vi "溶解氧电极校准.vi"() -> ()   [LabVIEW 2016, in "斯坦道多参数.lvlib"]
uses:
  <vilib>/Utility/miscctls.llb/LVPointTypeDef.ctl
  <vilib>/Analysis/NI_AALBase.lvlib
panel:
  out "滤波设定":dbl
  out "标液2":string="饱和标准液"
  out "标液1":string="零点标准液"
  in  "刷新按钮":bool
  out "第二点信号值":dbl
  out "第一点信号值":dbl
  out "通讯状态":string
  out "第二点校准值":dbl
  out "第一点校准值":dbl
  out "最小值":sgl format="%#.2f"
  out "最大值":sgl format="%#.2f"
  in  "校准模式":u16(ring)=1 items=["两点校准", "单点校准"]
  in  "校准停止":bool
  in  "校准启动":bool
  out "波形图表":sgl(graph) caption="历史曲线"
  out "变异系数":dbl format="%#.6f"
  out "standard deviation":dbl caption="标准差" format="%#.2f"
  out "mean":dbl caption="均值" format="%#.2f"
  out "测量读值":dbl caption="测量值" format="%#.2f"
  out "偏移值补偿":dbl caption="溶解氧偏移修正值" format="%#.2f"
  out "饱和度值":dbl format="%#.2f"
  out "提示":string
  out "气压补偿值":dbl format="%#.2f"
  out "盐度补偿值":dbl format="%#.2f"
  out "电极斜率":dbl format="%#.6f"
  out "电极零点":dbl format="%#.6f"
  # "溶解氧电极设定"
  # "%"
  # "%"
  # "ppt"
  # "hPa"
  # "请选择校准模式:"
  # "mg/L"
  # "%"
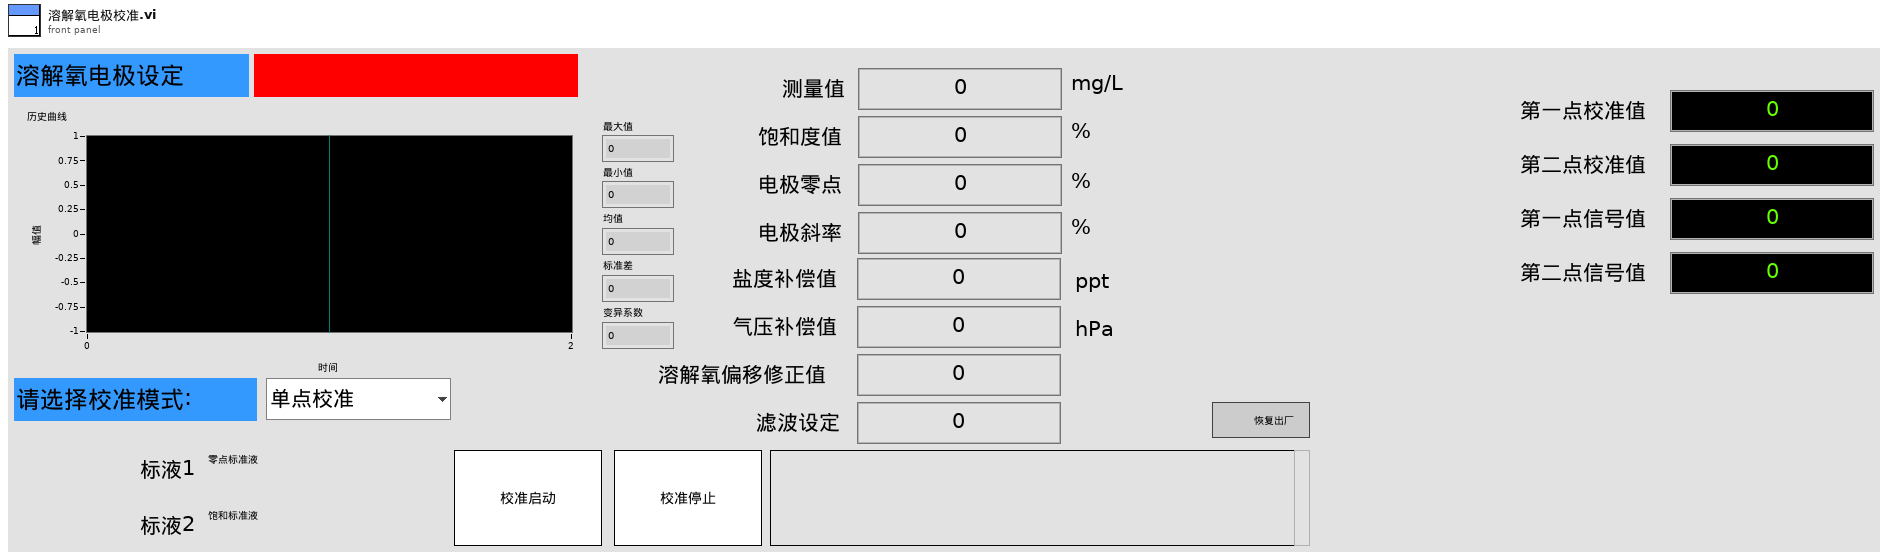
[diagram p1: front panel]
types:
  T1 = typedef "LVPointTypeDef.ctl" = cluster{"Horizontal":i16, "Vertical":i16}
  T2 = cluster{"电极状态标志":u16, "电极型号标志":u16, "溶解氧测量值":sgl, "温度测量值":sgl, "溶解氧饱和度值":sgl, "盐度补偿值":sgl, "大气压补偿值":sgl, "溶解氧偏移修正值":sgl, "温度偏移修正值":sgl, "手动温度补偿值":sgl, "溶解氧电极零点":sgl, "溶解氧电极斜率":sgl, "第1点标准值记录":sgl, "第1点信号值记录":sgl, "第1点温度值记录":sgl, "第2点标准值记录":sgl, "第2点信号值记录":sgl, "第2点温度值记录":sgl, "命令滤波设定":u16, "温度模式":enum16{"ATC", "MTC"}, "生产批次":u16, "电极序号":u16, "串口地址":u16, "串口波特率":enum16{"9600", "19200", "115200"}, "串口校验位":enum16{"NONE", "ODD", "EVEN"}, "串口停止位":enum16{"1bit", "2bit"}, "第一点标准值":sgl, "第二点标准值":sgl}
  T3 = enum8{"Enabled", "Disabled", "Disabled and Grayed Out"}
  T4 = cluster{"测量量程":dbl, "测量精度":dbl, "测量间隔":dbl, "消解温度":dbl, "消解时长":dbl, "空白校准时间":timestamp, "曲线截距":dbl, "曲线斜率":dbl, "测量检出限":dbl, "测量信号值":dbl, "线性相关系数":dbl, "二次多项式系数":dbl, "标样校准时间":timestamp, "单位":enum16{"ug/L", "mg/L"}}
  T5 = cluster{"ph":bool, "DO":bool, "Cond":bool, "Turb":bool, "叶绿素a":bool, "藻密度":bool, "ORP":bool}
  T6 = cluster{"温度测量值":sgl, "测量值":sgl, "温度偏移修正值":sgl, "信号值":sgl}
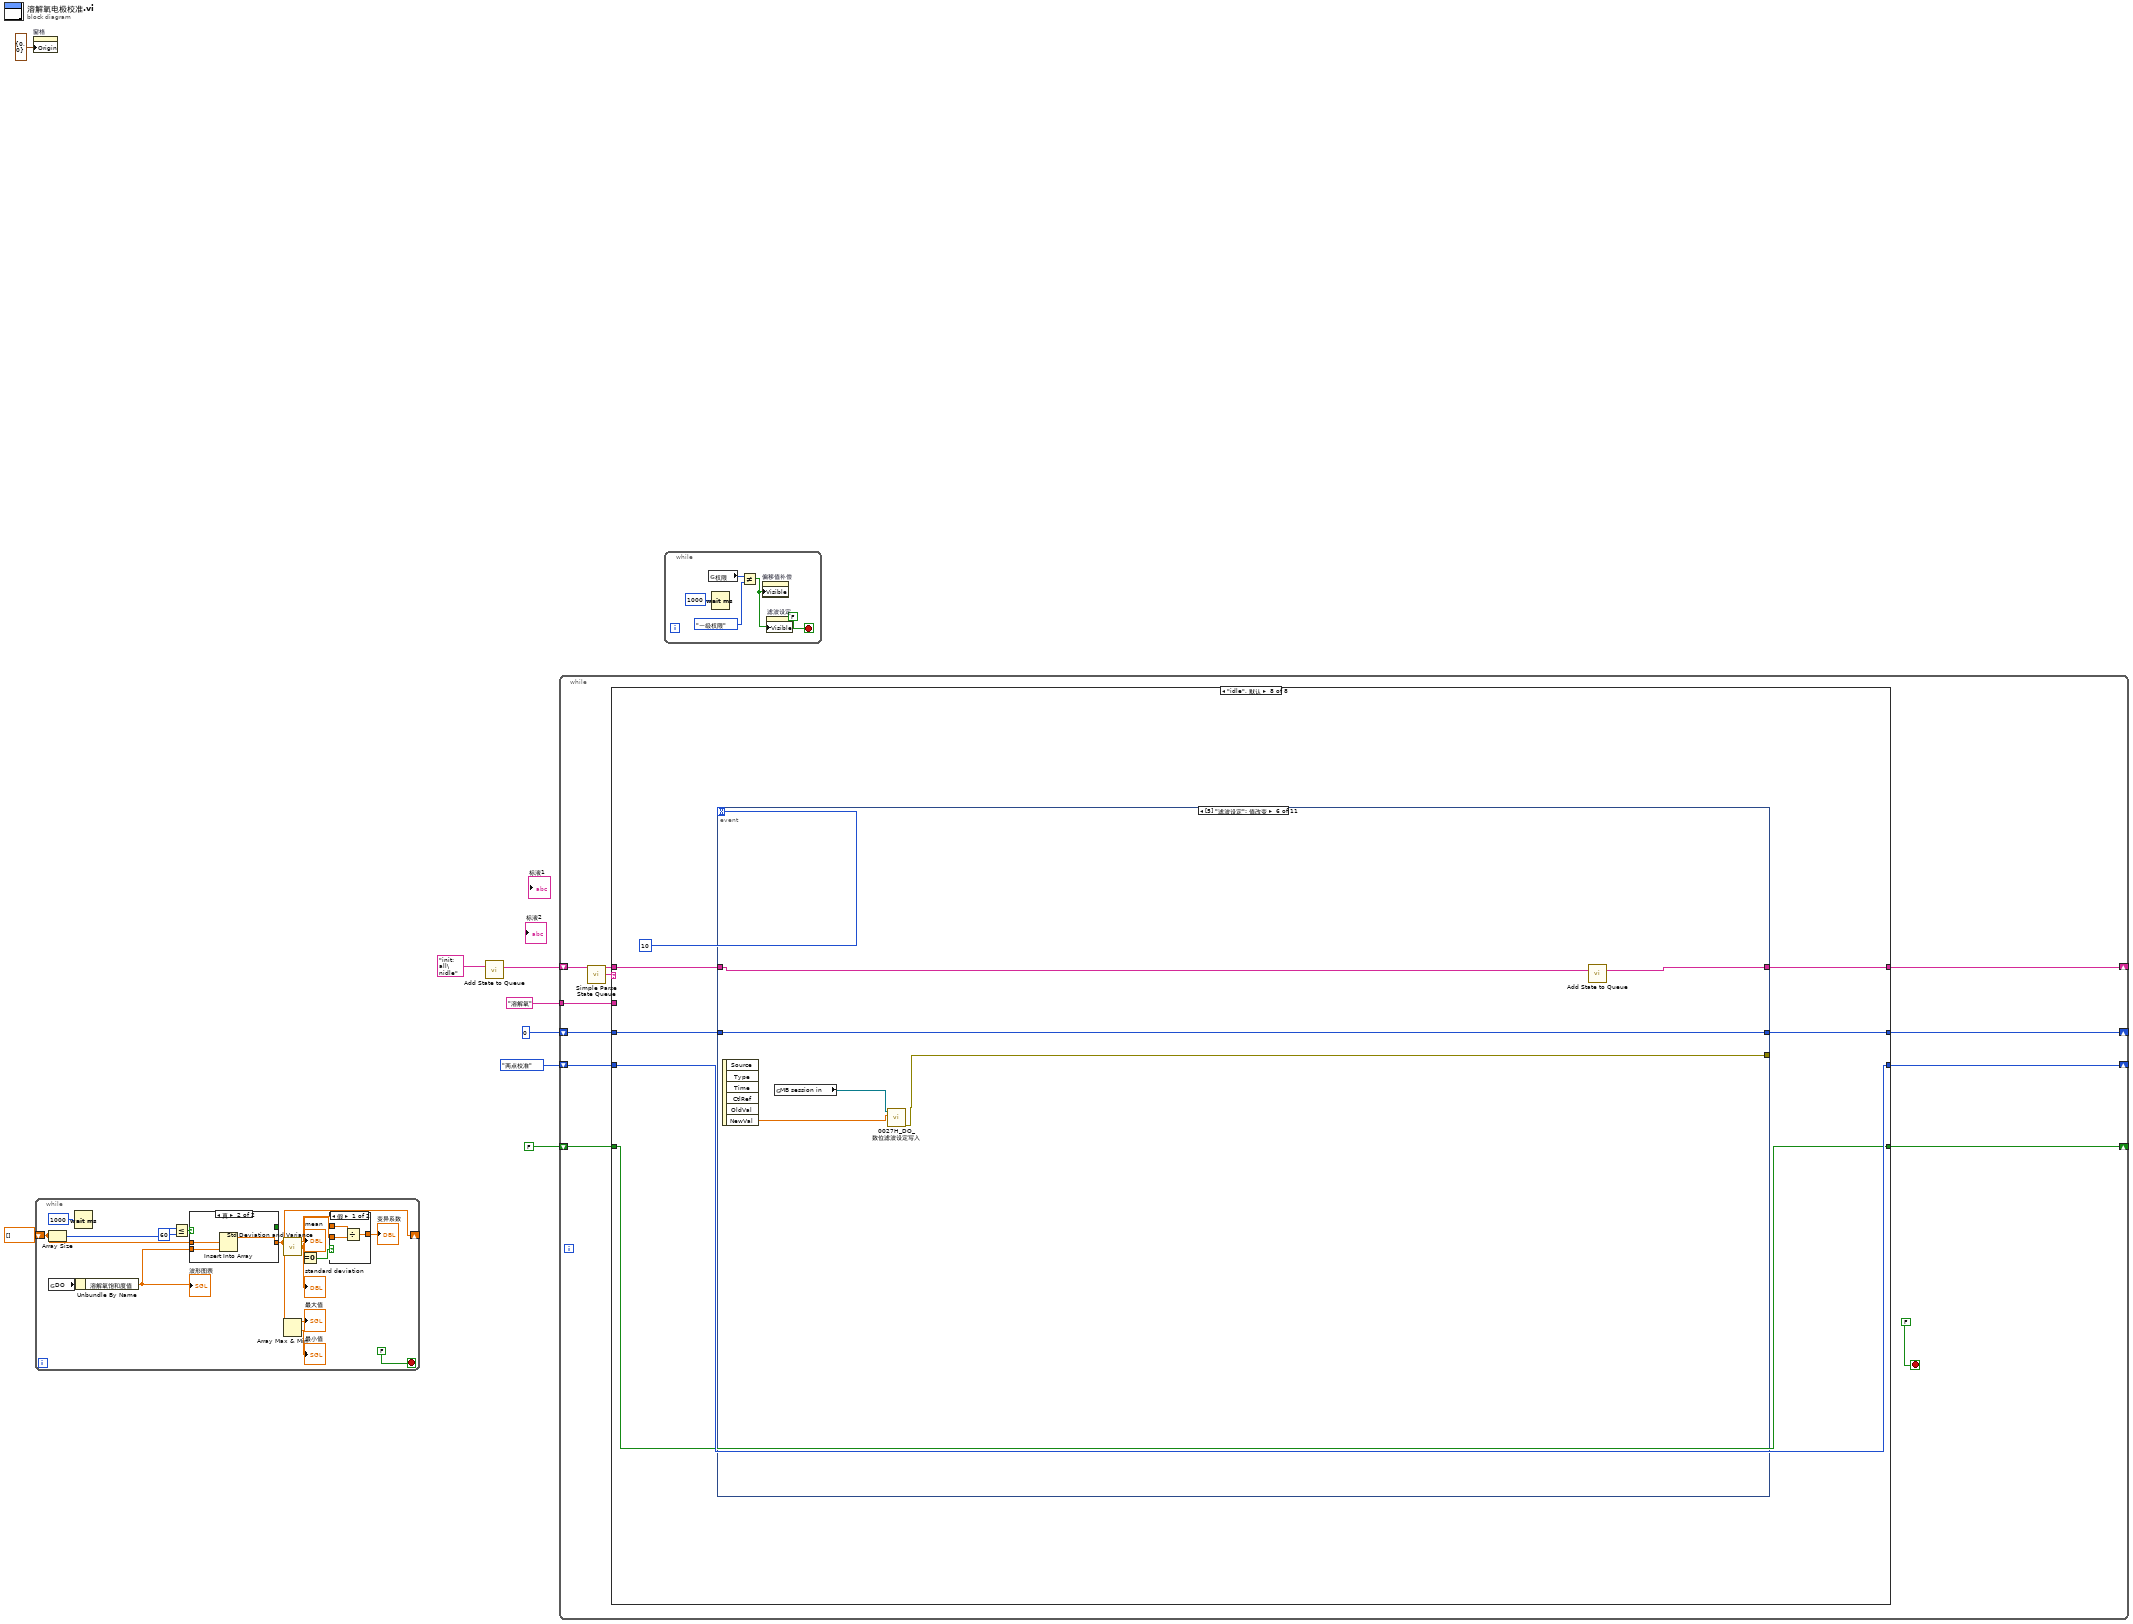
[diagram p0: block diagram]
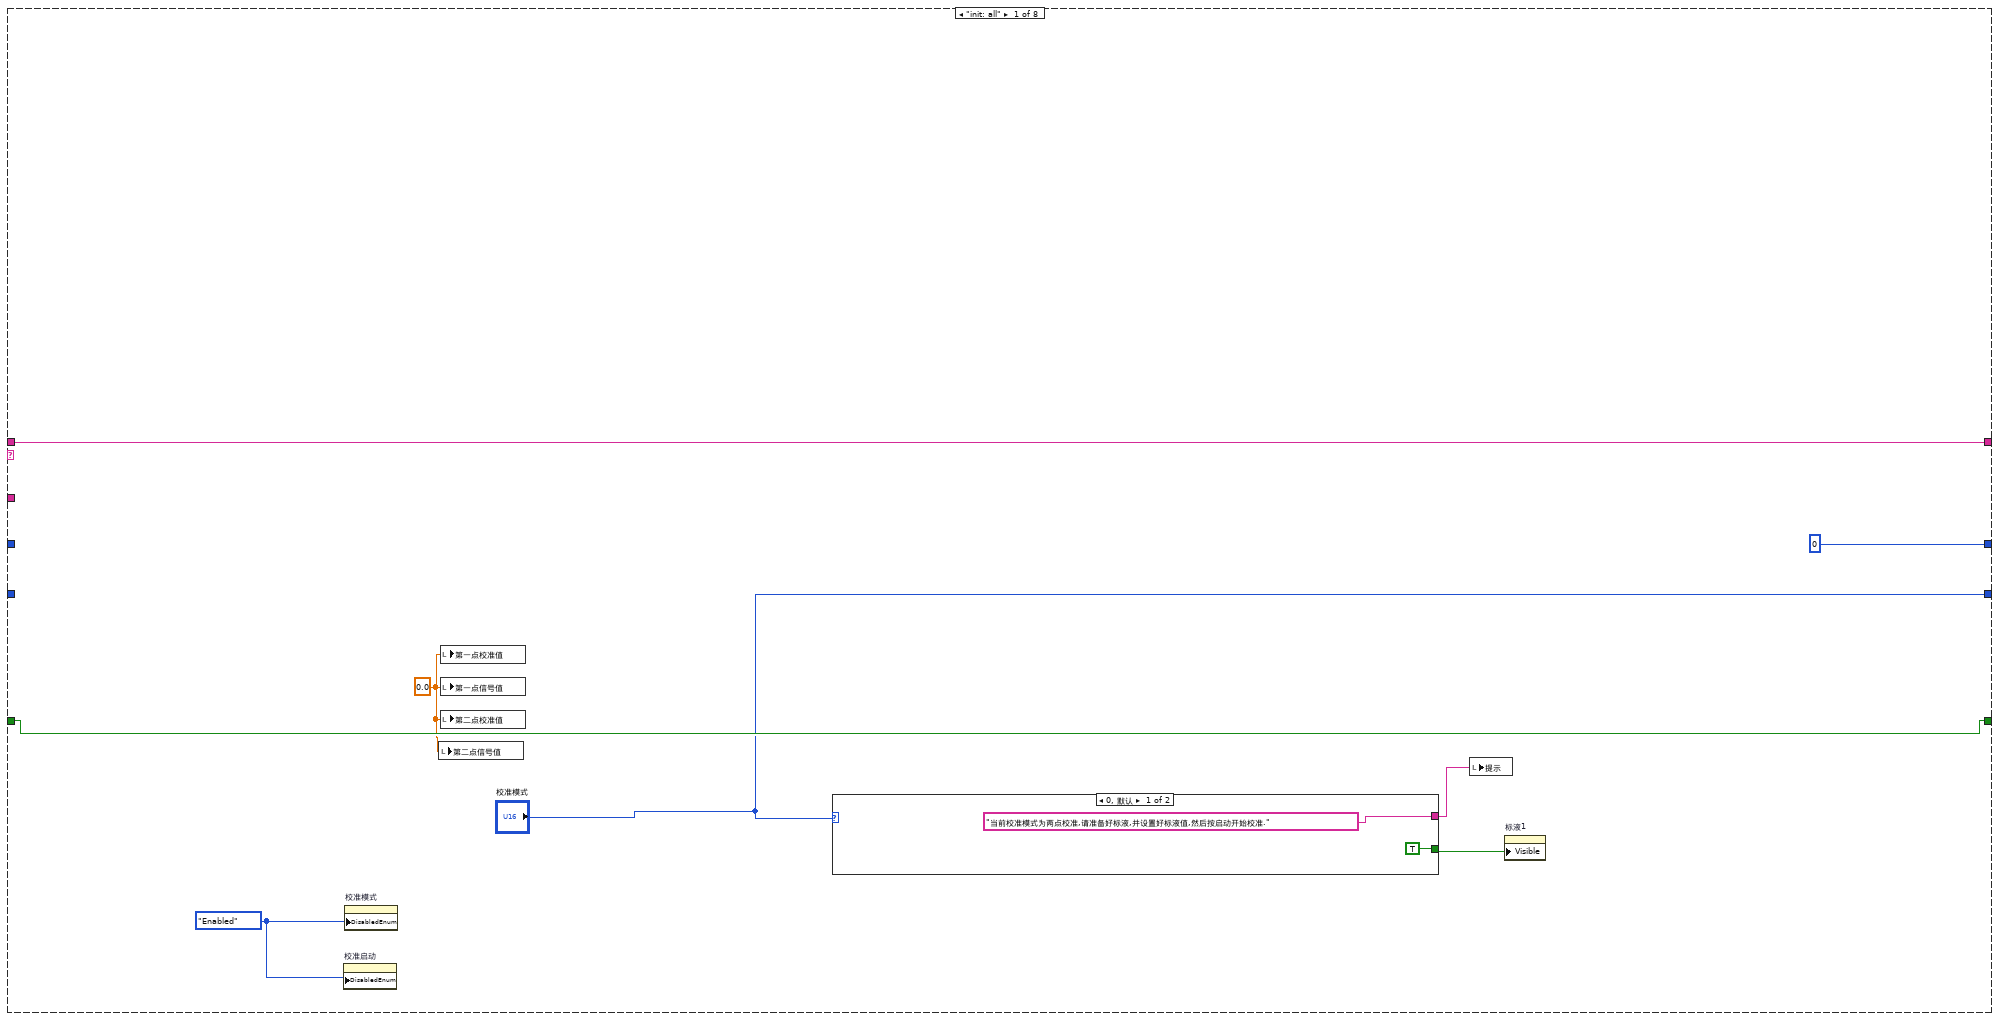
[diagram p2: hidden frame]
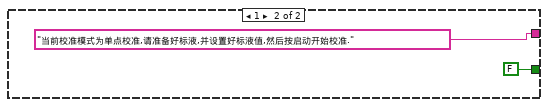
[diagram p3: hidden frame]
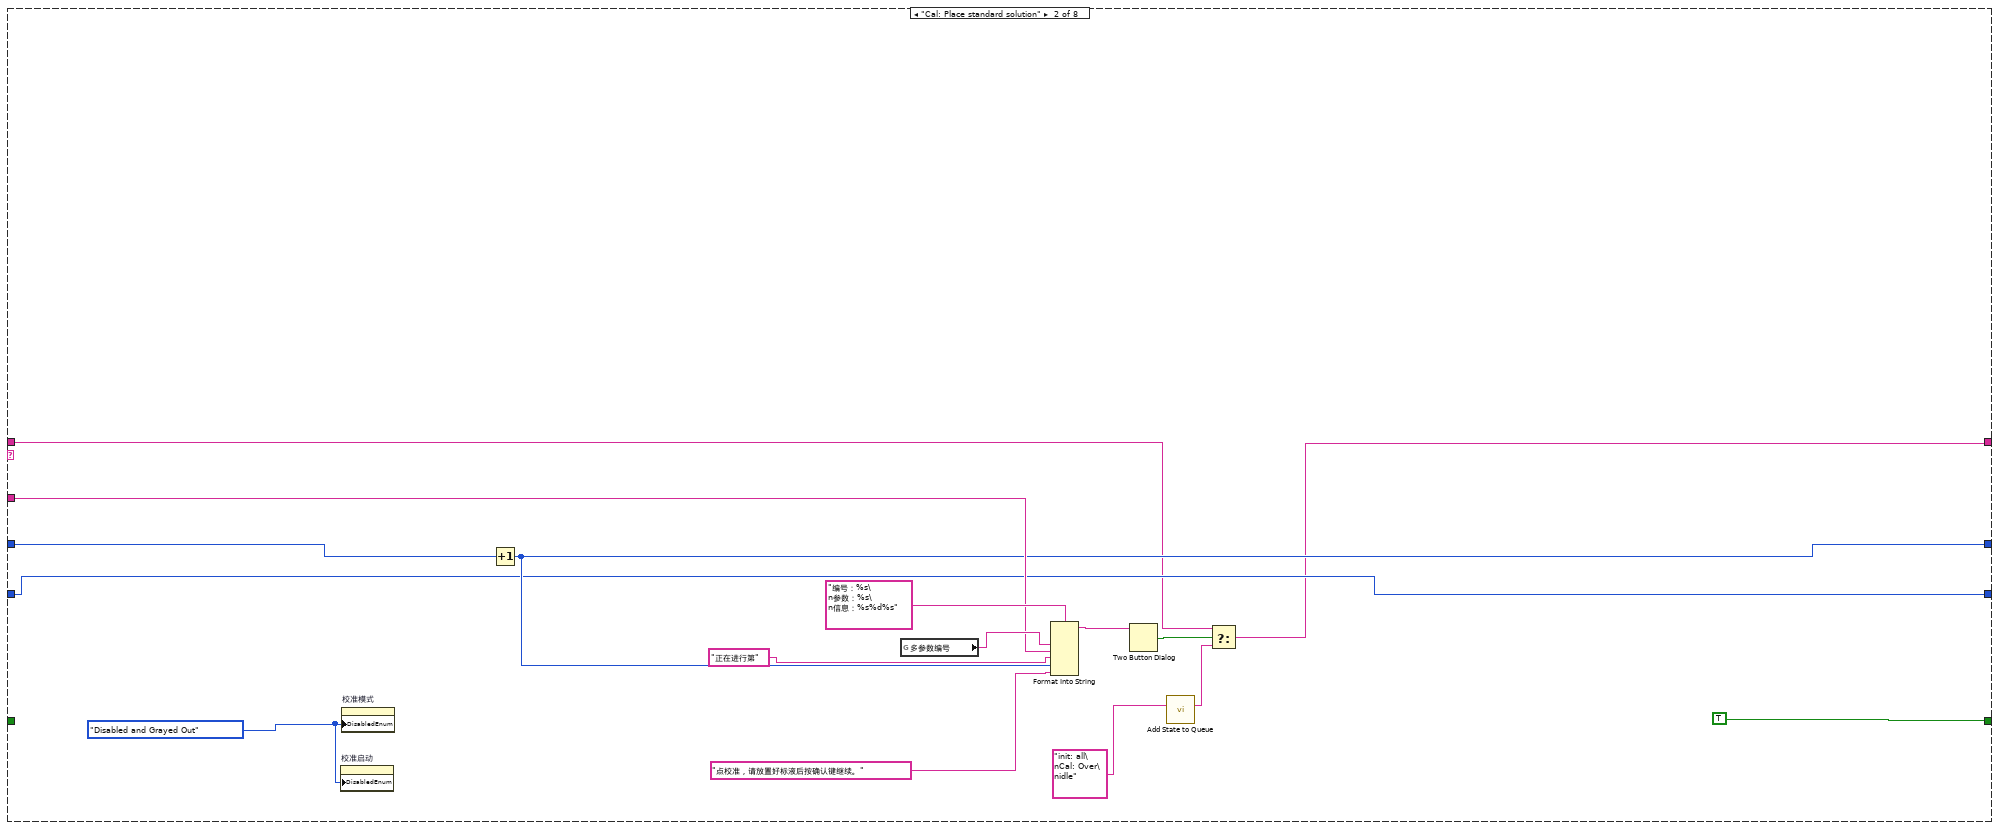
[diagram p4: hidden frame]
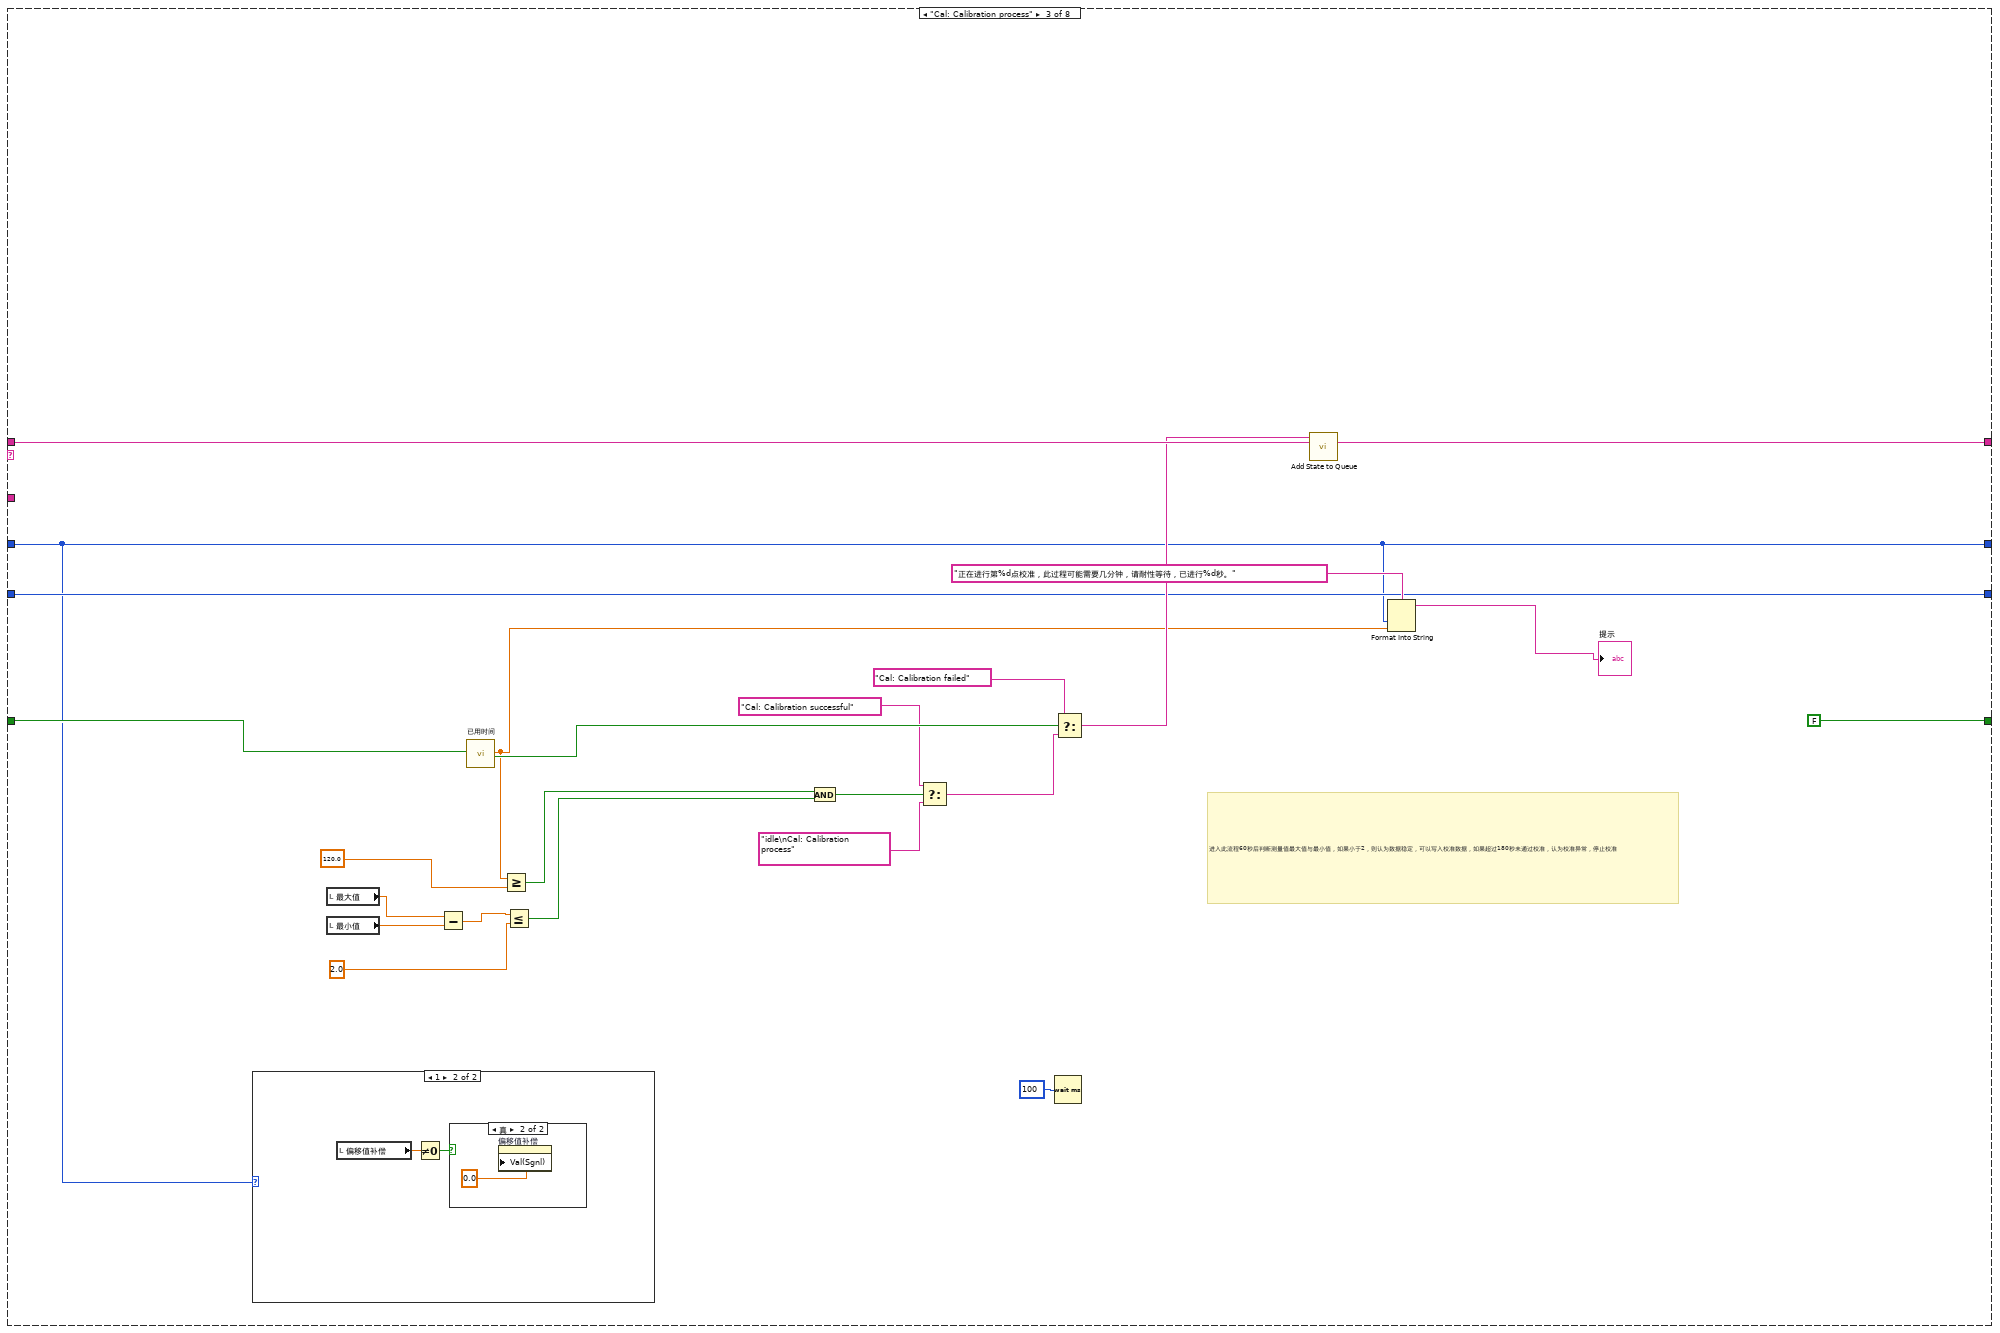
[diagram p5: hidden frame]
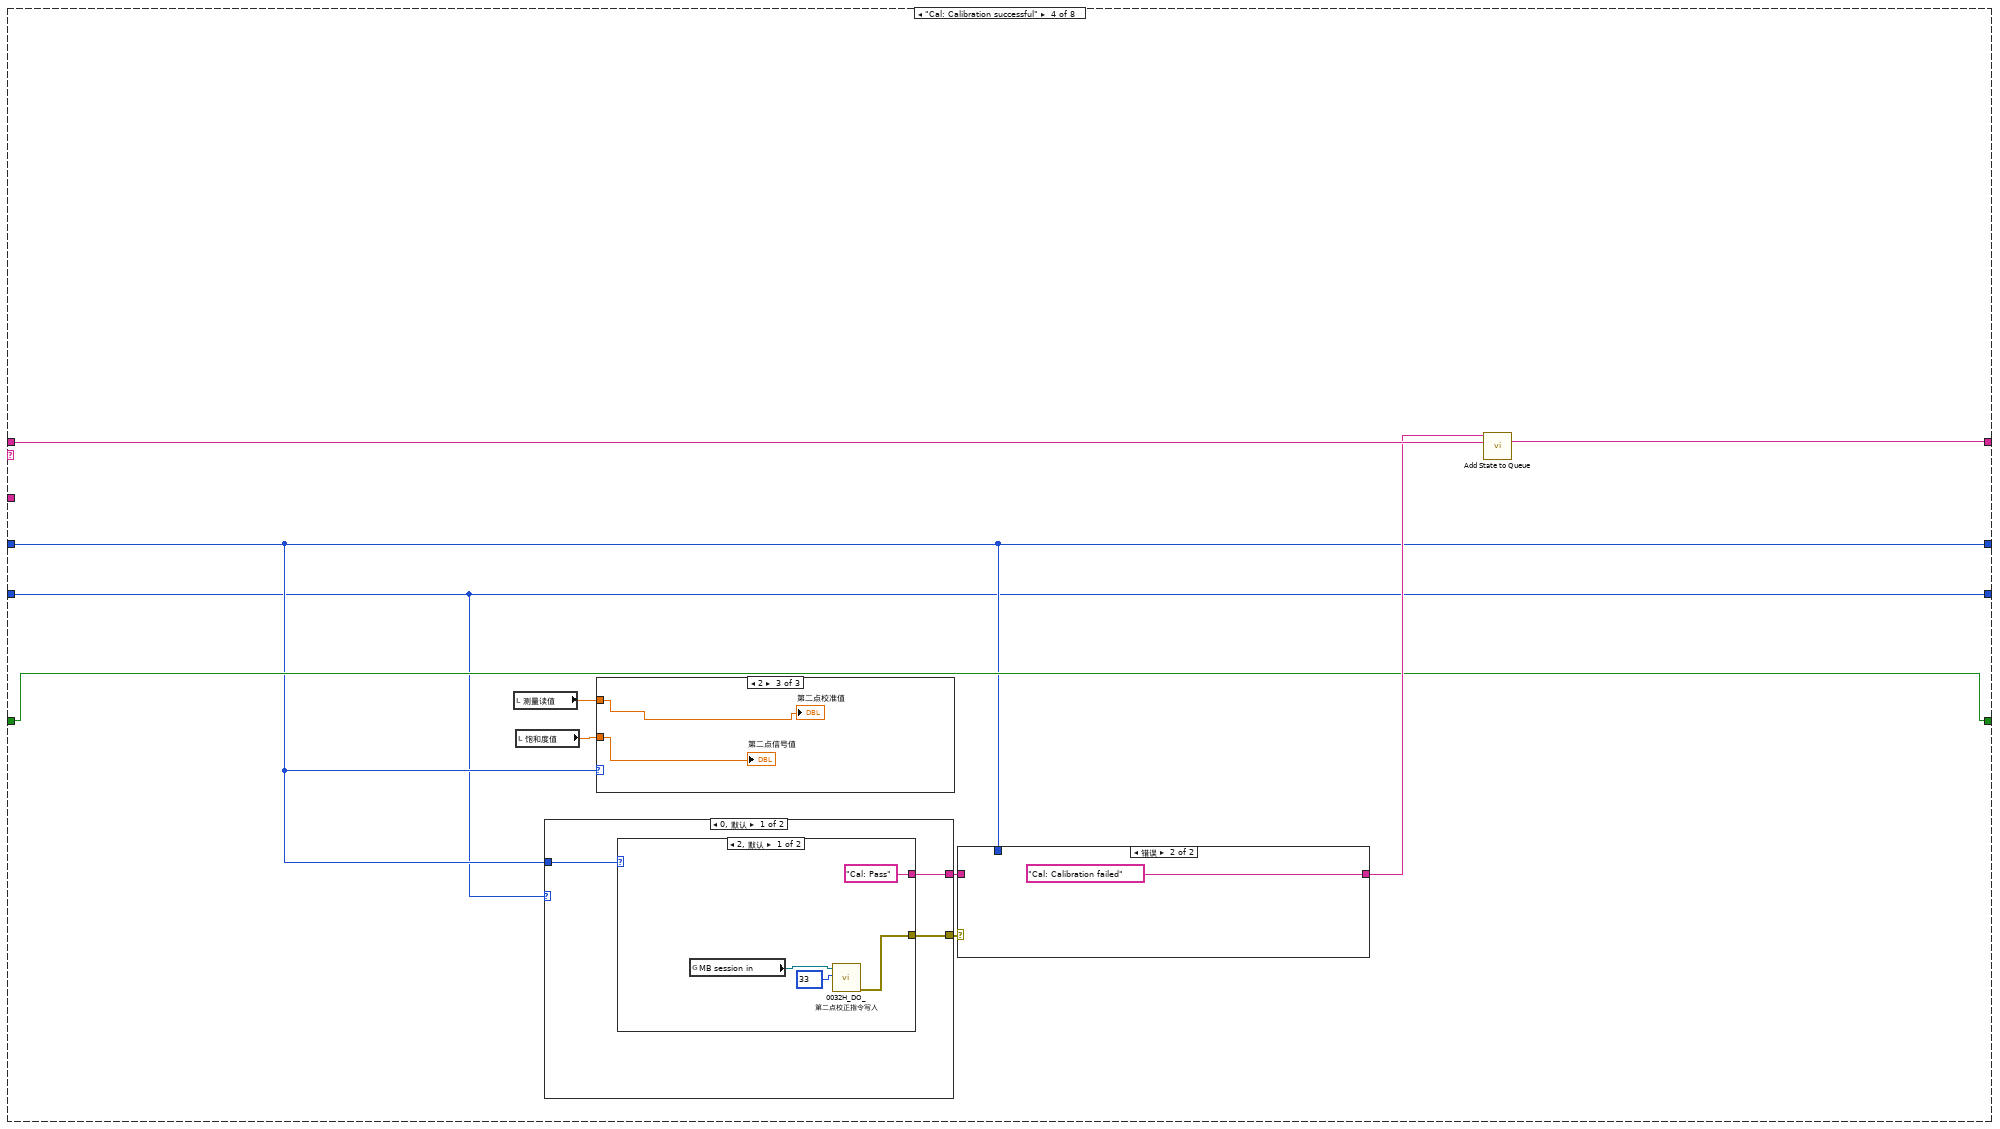
[diagram p8: hidden frame]
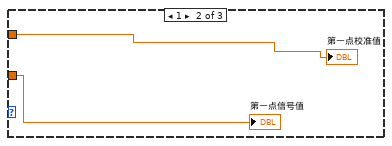
[diagram p10: hidden frame]
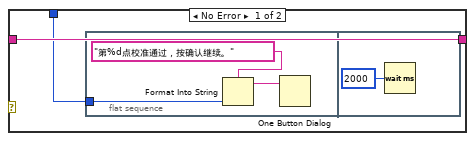
[diagram p11: hidden frame]
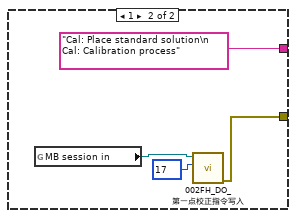
[diagram p12: hidden frame]
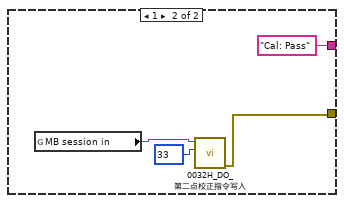
[diagram p13: hidden frame]
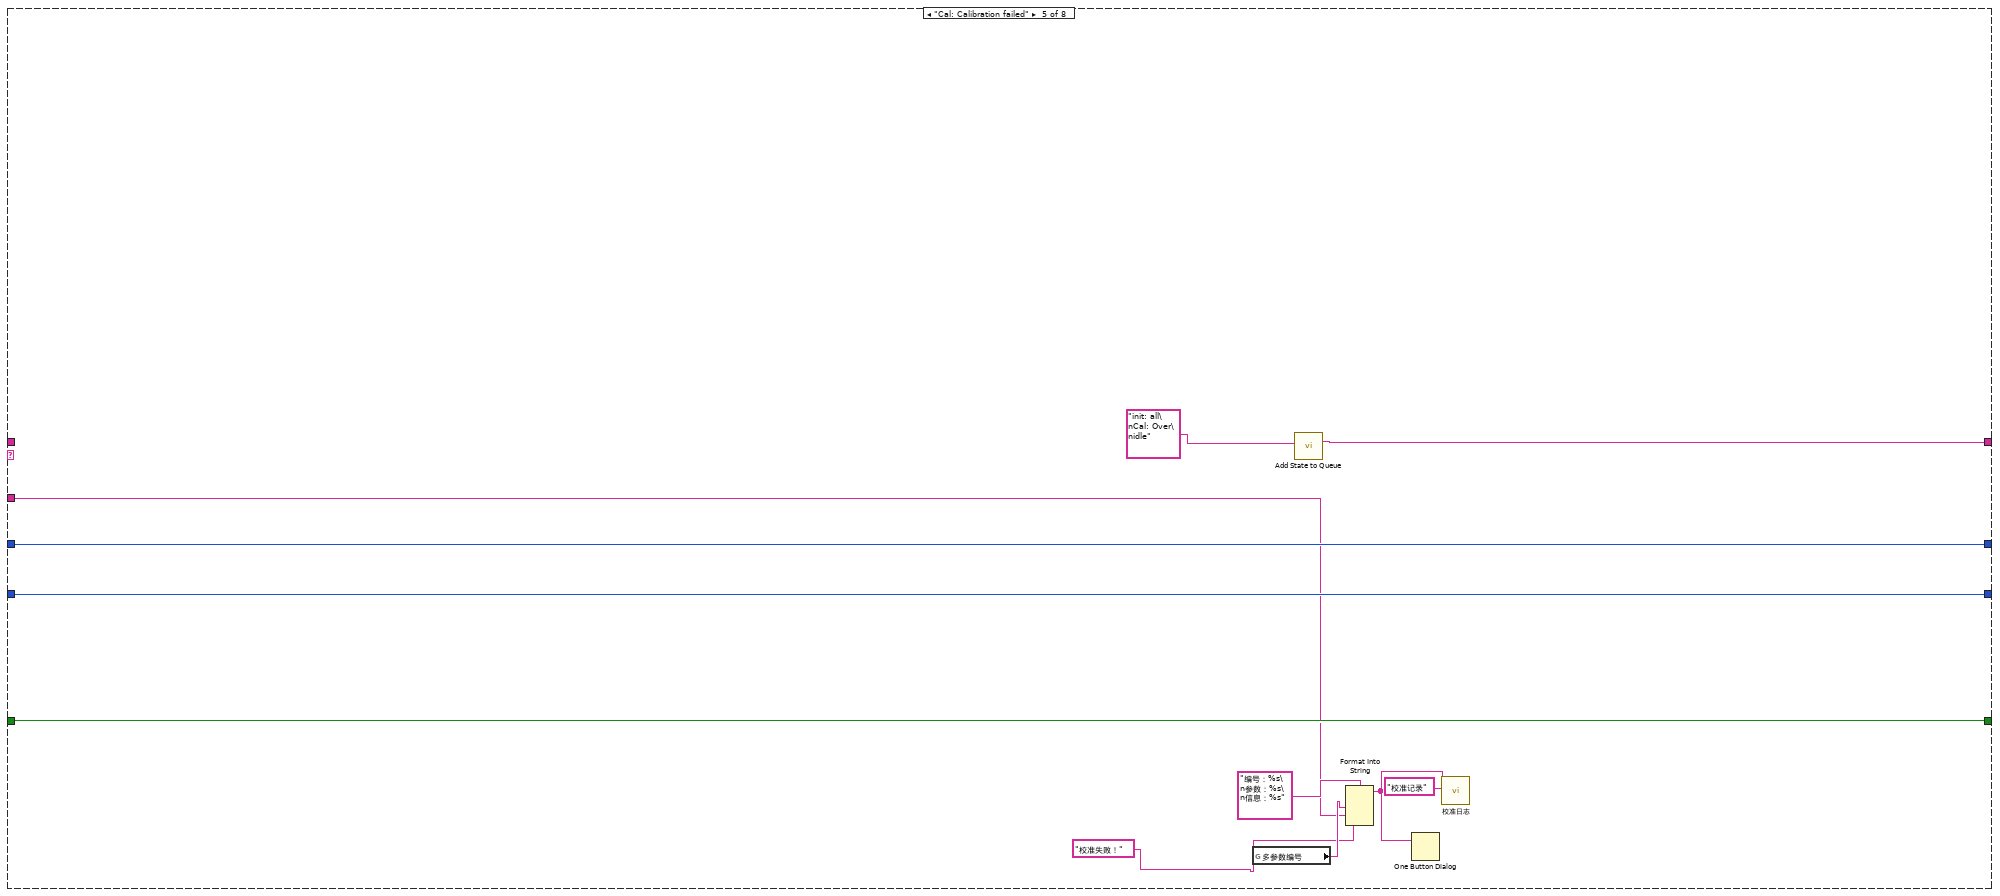
[diagram p14: hidden frame]
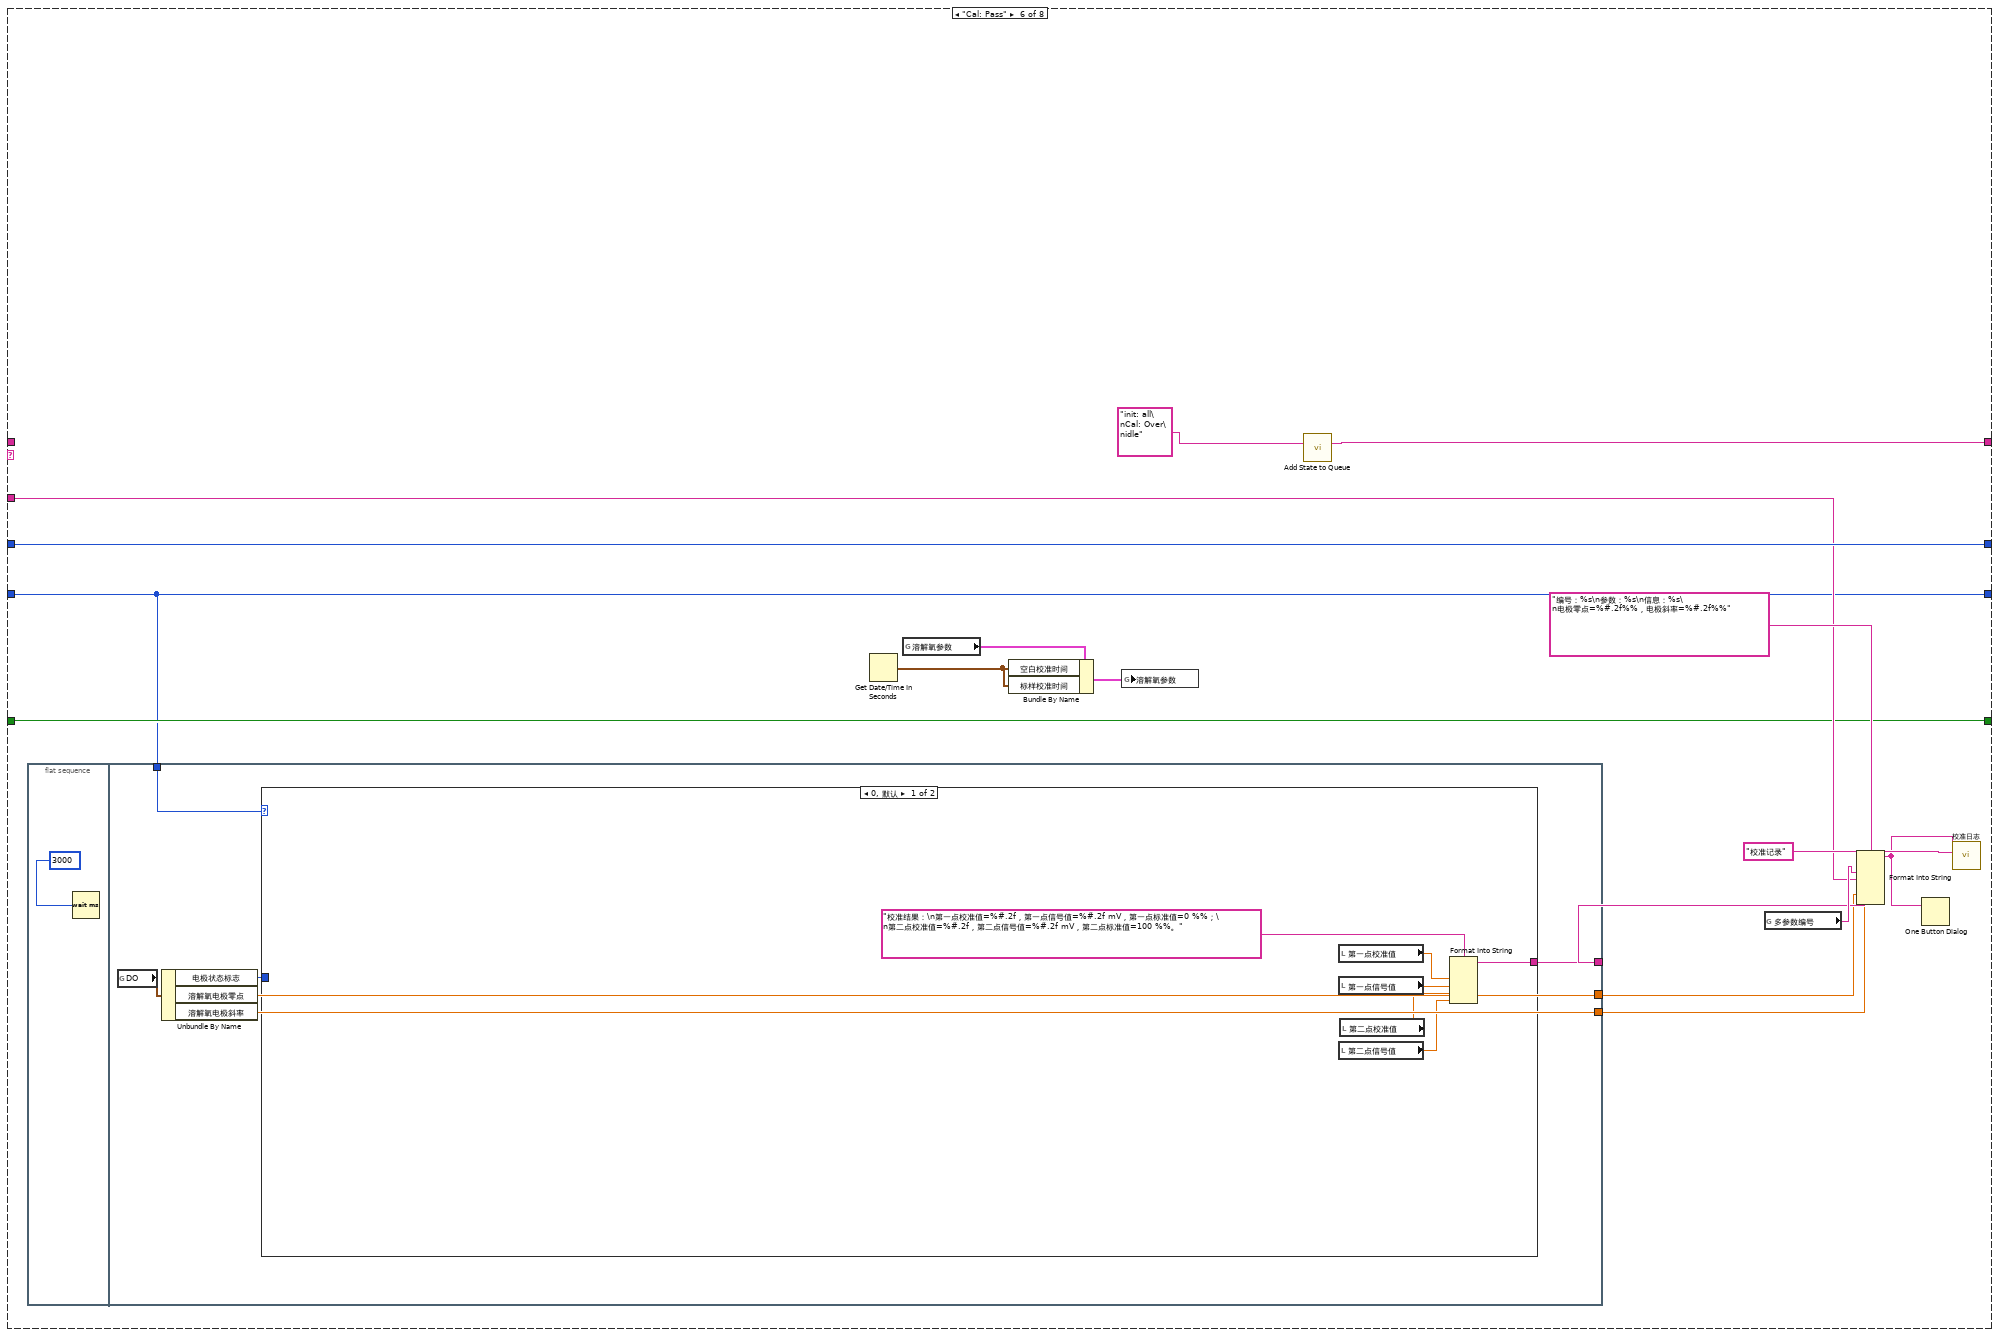
[diagram p15: hidden frame]
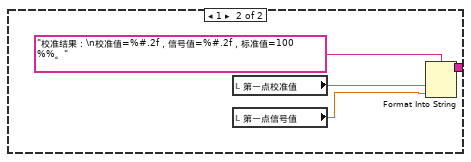
[diagram p16: hidden frame]
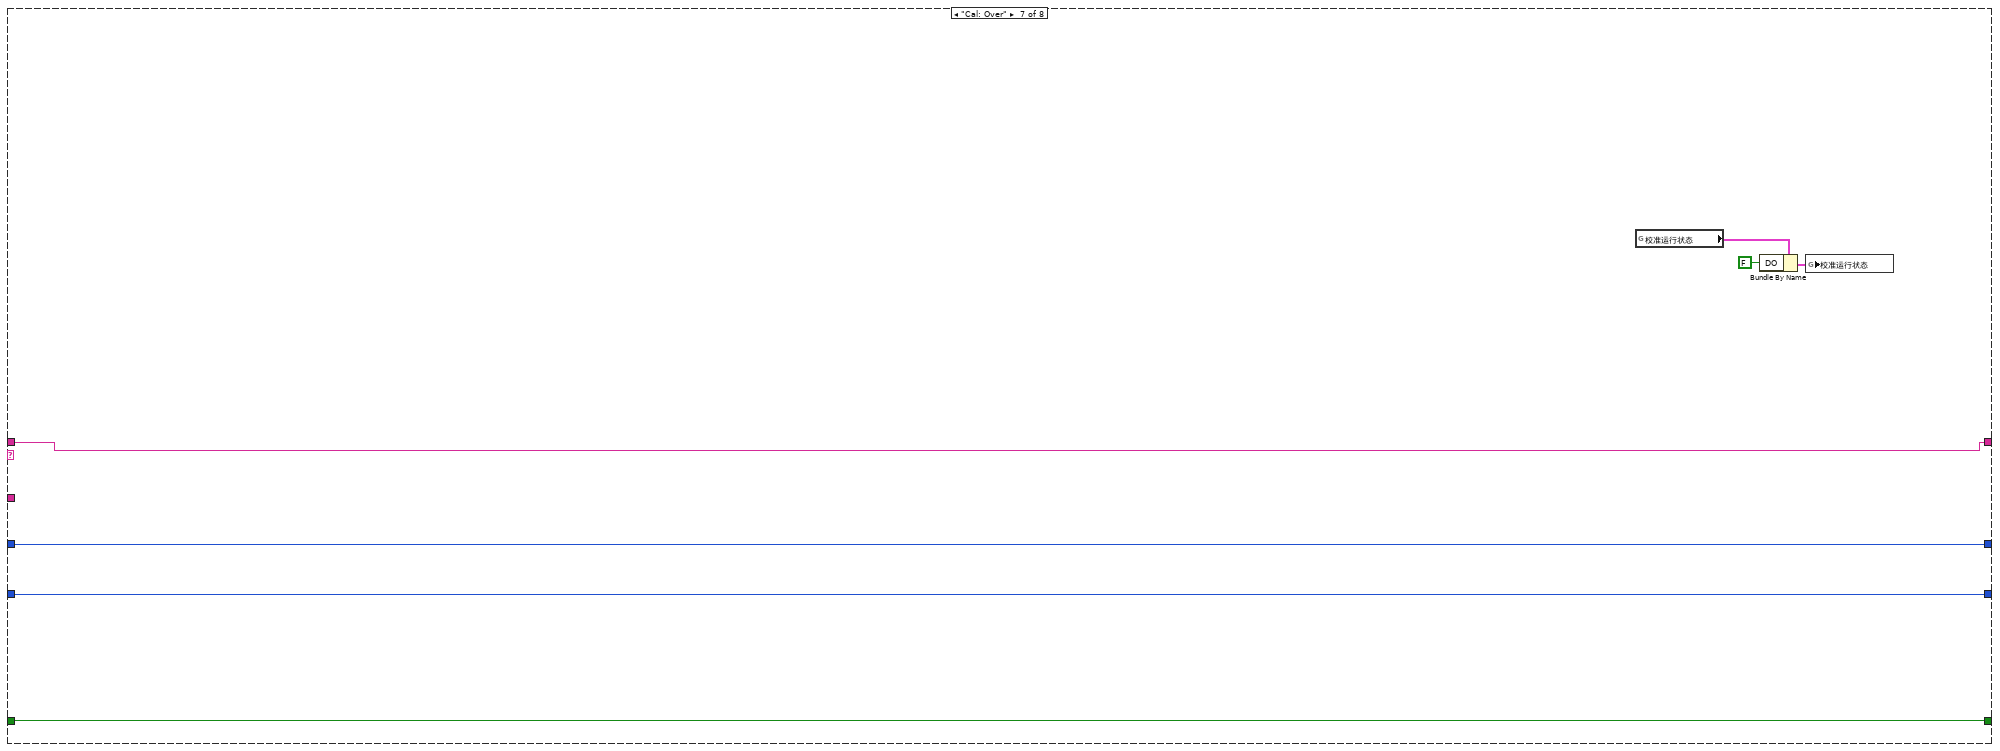
[diagram p17: hidden frame]
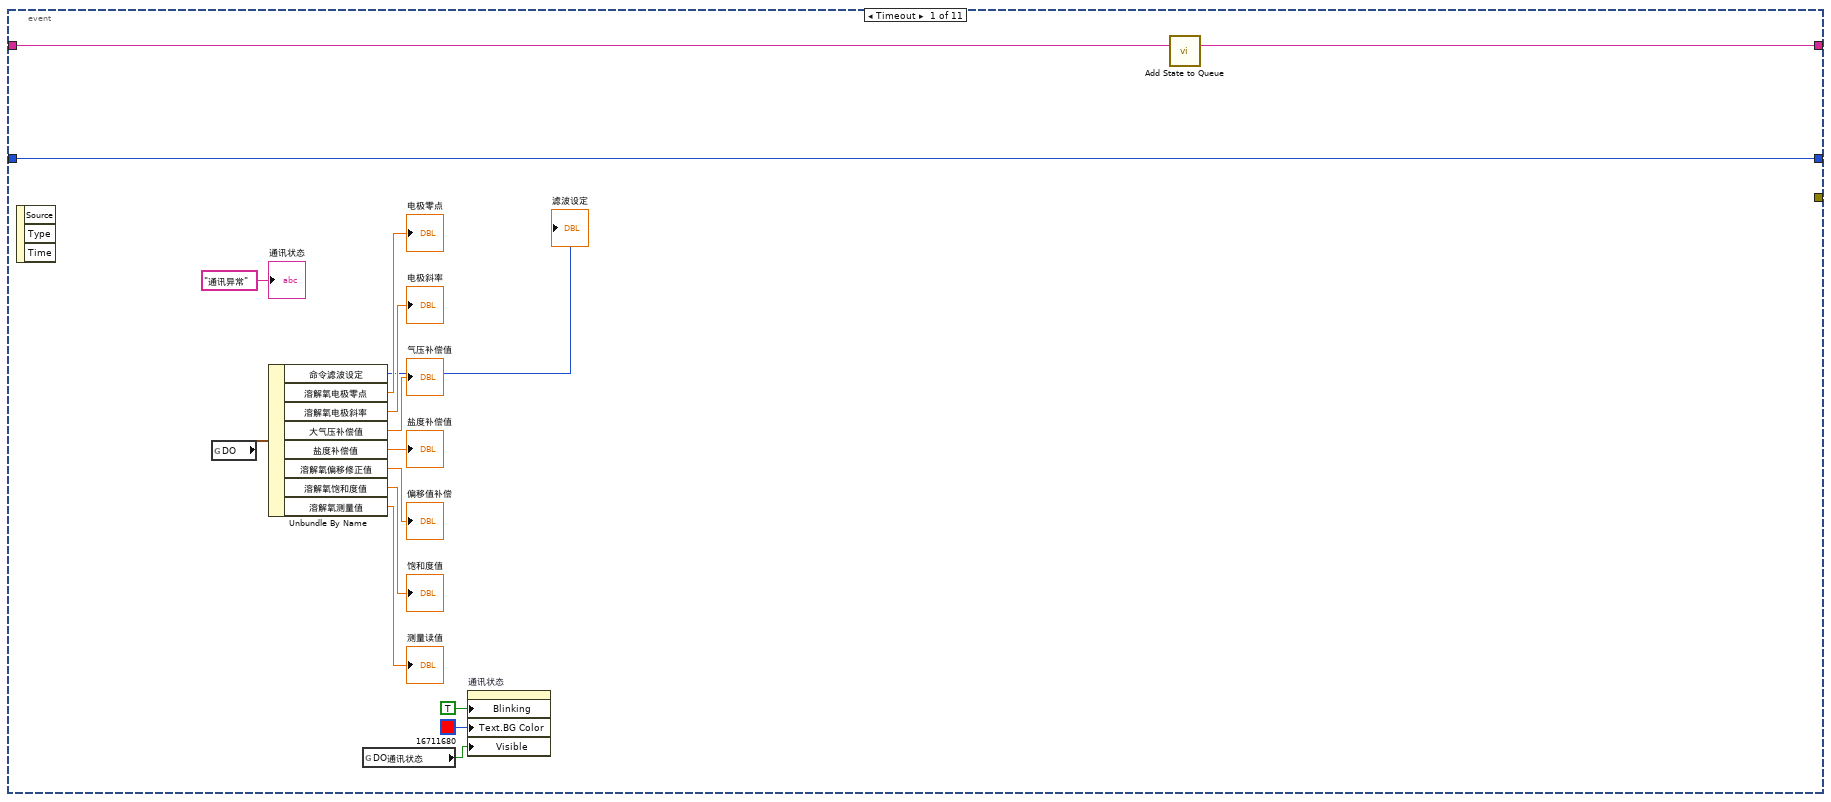
[diagram p18: hidden frame]
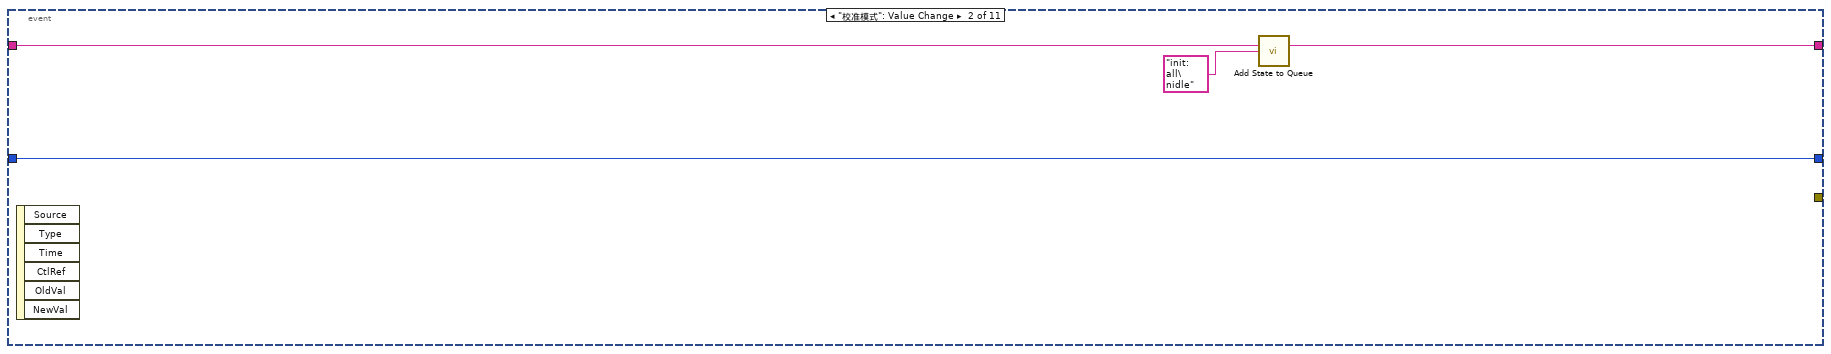
[diagram p19: hidden frame]
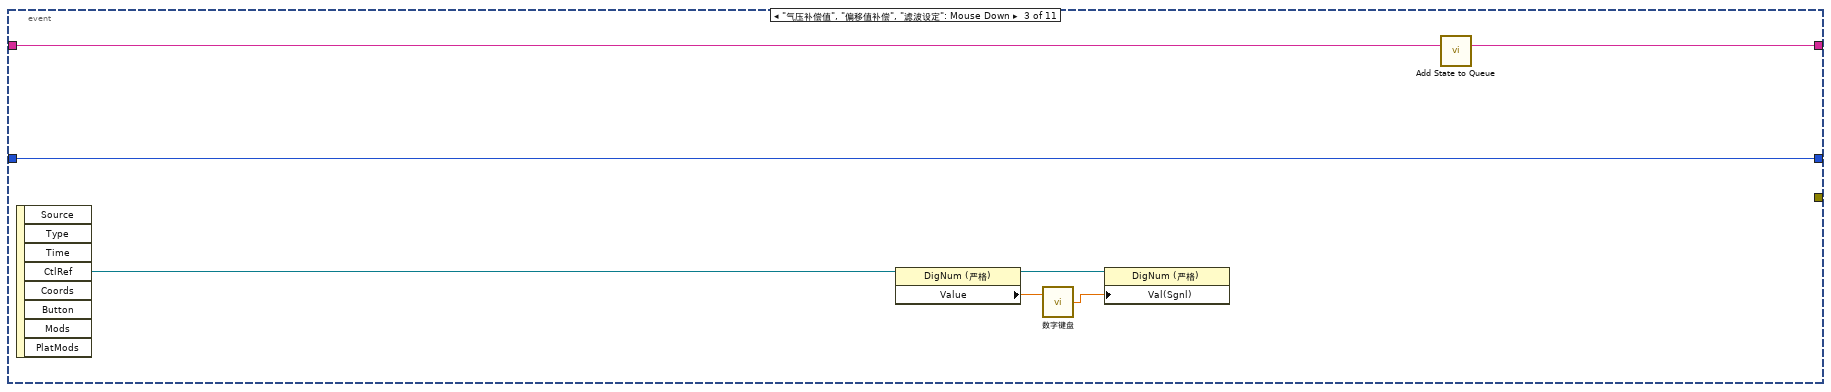
[diagram p20: hidden frame]
diagram:
  n1 = property on="窗格" class="Pane"("Origin"=T1 {"Horizontal"=0, "Vertical"=0} ("原点")) -> ()  [unwired: 2 in, 2 out]
  n2 = while {
    shift-right: [w12] -> _
    shift-left: sgl[] [] -> [w19]
    stop <- FALSE stop-if-true
    n3 = Array Size(array=w19) -> (size(s)=w21:i32)
    n4 = global read "国弘过程全局变量.vi" "DO"() -> (w15:T2)
    n5 = Wait (ms)(milliseconds to wait=u32 1000 ("等待时间（毫秒）")) -> ()  [unwired: 1 out]
    n6 = Unbundle By Name(w15) -> ("溶解氧饱和度值"=w9:sgl)
    "波形图表" <- w9
    n7 = Less Or Equal?(x=w21, y=60) -> (x <= y?=w20:bool)
    n8 = case shown="真" w20 {
      tunnel: w19 -> [w32 w35]
      tunnel: w9 -> [w30 w34]
      tunnel: [w28 w33] -> w12
      tunnel: [TRUE _] -> _
      frame False {
        n9 = Replace Array Subset(array=w32, new element=w30) -> (w31:sgl[])  [unwired: 1 in]
        n10 = Rotate 1D Array(1:w31, 2:-1 ("n")) -> (0:w28:sgl[])
      }
      frame True {
        n11 = Insert Into Array(array=w35, new element=w34) -> (w33:sgl[])  [unwired: 1 in]
      }
    }
    n12 = call <vilib>:"Std Deviation and Variance.vi"("X"=w12) -> ("mean"=w14:dbl, "standard deviation"=w13:dbl)  [unwired: 1 in, 1 out]
    "mean" <- w14
    "standard deviation" <- w13
    n13 = Array Max & Min(array=w12) -> (max value=→"最大值":sgl, min value=→"最小值":sgl)  [unwired: 2 out]
    n14 = Equal To 0?(x=w14) -> (x = 0?=w18:bool)
    n15 = case shown="假" w18 {
      tunnel: w13 -> [w26 _]
      tunnel: [w25 _] -> w17
      tunnel: w14 -> [w24 _]
      frame False {
        n16 = Divide(x=w26, y=w24) -> (x/y=w25:dbl)
      }
      frame True {
      }
    }
    "变异系数" <- w17
  }
  n17 = call "Add State to Queue.vi"("State(s) In (\"\")"="init: all\nidle" ("State(s) In (\"\")")) -> ("States Out"=w5:string)  [unwired: 14 in]
  n18 = while {
    shift-right: [w43] -> _
    shift-left: w5 -> [w47]
    shift-right: [w40] -> _
    shift-left: 0 -> [w42]
    tunnel: "溶解氧" ("State(s) In (\"\")") -> [w41]
    shift-right: [w38] -> _
    shift-left: enum16{"两点校准", "单点校准"}."两点校准" ("校准模式") -> [w39]
    shift-right: [w36] -> _
    shift-left: FALSE -> [w37]
    stop <- FALSE stop-if-true
    n19 = call "Simple Parse State Queue.vi"("State Queue"=w47) -> ("Remain States"=w44:string, "Next State"=w45:string)  [unwired: 13 in]
    n20 = case shown="\"idle\", 默认" w45 {
      tunnel: w44 -> [w55 w63 w94 w110 _ _ w189 w196]
      tunnel: [w55 w62 w93 w109 w146 w156 w189 w195] -> w43
      tunnel: w42 -> [_ w71 w78 w104 w149 w165 w188 w193]
      tunnel: w41 -> [_ w72 _ _ w140 w161 _ _]
      tunnel: [0 w69 w78 w104 w149 w165 w188 w194] -> w40
      tunnel: w39 -> [_ w68 w79 w103 w148 w157 w187 w192]
      tunnel: ["校准模式" w68 w79 w103 w148 w157 w187 w192] -> w38
      tunnel: w37 -> [w52 _ w81 w105 w147 w160 w186 w190]
      tunnel: [w52 TRUE FALSE w105 w147 w160 w186 w190] -> w36
      frame "init: all" {
        w50 = T3."Enabled" ("禁用")
        w51 = 0.0 ("第一点校准值")
        n21 = property on="校准启动" class="Bool"("DisabledEnum"=w50) -> ()  [unwired: 2 in, 2 out]
        n22 = property on="校准模式" class="Ring (严格)"("DisabledEnum"=w50) -> ()  [unwired: 2 in, 2 out]
        n23 = local write "第二点信号值"(w51) -> ()
        n24 = local write "第一点校准值"(w51) -> ()
        n25 = local write "第一点信号值"(w51) -> ()
        n26 = local write "第二点校准值"(w51) -> ()
        n27 = case shown="0, 默认" "校准模式" {
          tunnel: ["当前校准模式为两点校准,请准备好标液,并设置好标液值,然后按启动开始校准." ("提示") "当前校准模式为单点校准,请准备好标液,并设置好标液值,然后按启动开始校准." ("提示")] -> w54
          tunnel: [TRUE ("可见") FALSE ("可见")] -> w48
          frame 0, Default {
          }
          frame 1 {
          }
        }
        n28 = local write "提示"(w54) -> ()
        n29 = property on="标液1" class="Str"("Visible"=w48) -> ()  [unwired: 2 in, 2 out]
      }
      frame "Cal: Place standard solution" {
        w61 = T3."Disabled and Grayed Out" ("禁用")
        n30 = property on="校准启动" class="Bool"("DisabledEnum"=w61) -> ()  [unwired: 2 in, 2 out]
        n31 = property on="校准模式" class="Ring (严格)"("DisabledEnum"=w61) -> ()  [unwired: 2 in, 2 out]
        n32 = Increment(x=w71) -> (x+1=w69:i32)
        n33 = global read "多参数全局变量.vi" "多参数编号"() -> (w74:string)
        n34 = Format Into String(format string="编号：%s\n参数：%s\n信息：%s%d%s" ("格式字符串"), w74, w72, "正在进行第" ("消息"), w69, "点校准，请放置好标液后按确认键继续。" ("消息")) -> (resulting string=w66:string)  [unwired: 2 in, 1 out]
        n35 = Two Button Dialog(message=w66) -> (T button?=w65:bool)  [unwired: 2 in]
        n36 = call "Add State to Queue.vi"("State(s) In (\"\")"="init: all\nCal: Over\nidle" ("State(s) In (\"\")")) -> ("States Out"=w64:string)  [unwired: 14 in]
        n37 = Select(t=w63, s=w65, f=w64) -> (s? t:f=w62:string)
      }
      frame "Cal: Calibration process" {
        # "进入此流程60秒后判断测量值最大值与最小值，如果小于2，则认为数据稳定，可以写入校准数据，如果超过180秒未通过校准，认为校准异常，停止校准"
        n38 = case shown="1" w78 {
          frame 0, Default {
          }
          frame 1 {
            n39 = local read "偏移值补偿"() -> (w100:dbl)
            n40 = Not Equal To 0?(x=w100) -> (x != 0?=w101:bool)
            n41 = case shown="真" w101 {
              frame False {
              }
              frame True {
                n42 = property on="偏移值补偿" class="DigNum (严格)"("Val(Sgnl)"=0.0 ("值(信号)")) -> ()  [unwired: 2 in, 2 out]
              }
            }
          }
        }
        n43 = local read "最大值"() -> (w98:sgl)
        n44 = local read "最小值"() -> (w97:sgl)
        n45 = Subtract(x=w98, y=w97) -> (x-y=w99:sgl)
        n46 = call "已用时间"("Reset"=w81) -> ("Elapsed Time (s)"=w77:dbl, "Time has Elapsed"=w95:bool)  [unwired: 11 in, 6 out]
        n47 = Greater Or Equal?(x=w77, y=120.0) -> (x >= y?=w90:bool)
        n48 = Less Or Equal?(x=w99, y=2.0) -> (x <= y?=w86:bool)
        n49 = And(x=w90, y=w86) -> (x .and. y?=w87:bool)
        n50 = Select(t="Cal: Calibration successful" ("State(s) In (\"\")"), s=w87, f="idle\nCal: Calibration process" ("State(s) In (\"\")")) -> (s? t:f=w85:string)
        n51 = Wait (ms)(milliseconds to wait=u32 100 ("等待时间（毫秒）")) -> ()  [unwired: 1 out]
        n52 = Select(t="Cal: Calibration failed" ("State(s) In (\"\")"), s=w95, f=w85) -> (s? t:f=w84:string)
        n53 = call "Add State to Queue.vi"("State(s) In Front (\"\")"=w84, "State(s) In (\"\")"=w94) -> ("States Out"=w93:string)  [unwired: 13 in]
        n54 = Format Into String(format string="正在进行第%d点校准，此过程可能需要几分钟，请耐性等待，已进行%d秒。" ("格式字符串"), w78, w77) -> (resulting string=→"提示":string)  [unwired: 2 in, 1 out]
      }
      frame "Cal: Calibration successful" {
        n55 = local read "测量读值"() -> (w106:dbl)
        n56 = local read "饱和度值"() -> (w107:dbl)
        n57 = case shown="0, 默认" w103 {
          tunnel: [w126 w135] -> w112
          tunnel: [w125 "Cal: Pass" ("State(s) In (\"\")")] -> w111
          tunnel: w104 -> [w124 _]
          frame 0, Default {
            n58 = case shown="2, 默认" w124 {
              tunnel: [w127 w131] -> w126
              tunnel: ["Cal: Pass" ("State(s) In (\"\")") "Cal: Place standard solution\n Cal: Calibration process" ("State(s) In (\"\")")] -> w125
              frame 2, Default {
                n59 = global read "多参数全局变量.vi" "MB session in"() -> (w128:refnum<class "MB_Master.lvclass">)
                n60 = call "0032H_DO_第二点校正指令写入.vi"("数值"=u16 33, "MB session in"=w128) -> ("error out"=w127:errorcluster)  [unwired: 8 in, 1 out]
              }
              frame 1 {
                n61 = global read "多参数全局变量.vi" "MB session in"() -> (w132:refnum<class "MB_Master.lvclass">)
                n62 = call "002FH_DO_第一点校正指令写入.vi"("数值"=u16 17, "MB session in"=w132) -> ("error out"=w131:errorcluster)  [unwired: 8 in, 1 out]
              }
            }
          }
          frame 1 {
            n63 = global read "多参数全局变量.vi" "MB session in"() -> (w137:refnum<class "MB_Master.lvclass">)
            n64 = call "0032H_DO_第二点校正指令写入.vi"("数值"=u16 33, "MB session in"=w137) -> ("error out"=w135:errorcluster)  [unwired: 8 in, 1 out]
          }
        }
        n65 = case shown="2" w104 {
          tunnel: w107 -> [_ w114 w116]
          tunnel: w106 -> [_ w113 w115]
          frame 0, Default {
          }
          frame 1 {
            "第一点信号值" <- w114
            "第一点校准值" <- w113
          }
          frame 2 {
            "第二点信号值" <- w116
            "第二点校准值" <- w115
          }
        }
        n66 = case shown="错误" w112 {
          tunnel: w111 -> [w118 _]
          tunnel: [w118 "Cal: Calibration failed" ("State(s) In (\"\")")] -> w108
          tunnel: w104 -> [w117 _]
          frame No Error {
            n67 = flat-sequence {
              tunnel: w117 -> [w119]
              frame #0 {
                n68 = Format Into String(format string="第%d点校准通过，按确认继续。" ("格式字符串"), w119) -> (resulting string=w121:string)  [unwired: 2 in, 1 out]
                n69 = One Button Dialog(message=w121) -> ()  [unwired: 1 in, 1 out]
              }
              frame #1 {
                n70 = Wait (ms)(milliseconds to wait=u32 2000 ("等待时间（毫秒）")) -> ()  [unwired: 1 out]
              }
            }
          }
          frame Error {
          }
        }
        n71 = call "Add State to Queue.vi"("State(s) In Front (\"\")"=w108, "State(s) In (\"\")"=w110) -> ("States Out"=w109:string)  [unwired: 13 in]
      }
      frame "Cal: Calibration failed" {
        n72 = global read "多参数全局变量.vi" "多参数编号"() -> (w143:string)
        n73 = call "Add State to Queue.vi"("State(s) In (\"\")"="init: all\nCal: Over\nidle" ("State(s) In (\"\")")) -> ("States Out"=w146:string)  [unwired: 14 in]
        n74 = Format Into String(format string="编号：%s\n参数：%s\n信息：%s" ("格式字符串"), w143, w140, "校准失败！" ("消息")) -> (resulting string=w142:string)  [unwired: 2 in, 1 out]
        n75 = One Button Dialog(message=w142) -> ()  [unwired: 1 in, 1 out]
        n76 = call "校准日志.vi"("table"="校准记录", "日志信息"=w142) -> ()  [unwired: 9 in, 1 out]
      }
      frame "Cal: Pass" {
        n77 = flat-sequence {
          tunnel: [w170] -> w158
          tunnel: w157 -> [w169]
          tunnel: [w168] -> w155
          tunnel: [w167] -> w154
          frame #0 {
            n78 = Wait (ms)(milliseconds to wait=u32 3000 ("等待时间（毫秒）")) -> ()  [unwired: 1 out]
          }
          frame #1 {
            n79 = global read "国弘过程全局变量.vi" "DO"() -> (w171:T2)
            n80 = Unbundle By Name(w171) -> ("电极状态标志"=w172:u16, "溶解氧电极零点"=w168:sgl, "溶解氧电极斜率"=w167:sgl)
            n81 = case shown="0, 默认" w169 {
              tunnel: [w178 w182] -> w170
              tunnel: w172 -> [_ _]
              frame 0, Default {
                n82 = local read "第一点校准值"() -> (w176:dbl)
                n83 = local read "第一点信号值"() -> (w177:dbl)
                n84 = local read "第二点信号值"() -> (w173:dbl)
                n85 = local read "第二点校准值"() -> (w174:dbl)
                n86 = Format Into String(format string="校准结果：\n第一点校准值=%#.2f，第一点信号值=%#.2f mV，第一点标准值=0 %%；\n第二点校准值=%#.2f，第二点信号值=%#.2f mV，第二点标准值=100 %%。" ("提示"), w176, w177, w174, w173) -> (resulting string=w178:string)  [unwired: 2 in, 1 out]
              }
              frame 1 {
                n87 = local read "第一点校准值"() -> (w181:dbl)
                n88 = local read "第一点信号值"() -> (w179:dbl)
                n89 = Format Into String(format string="校准结果：\n校准值=%#.2f，信号值=%#.2f，标准值=100 %%。" ("提示"), w181, w179) -> (resulting string=w182:string)  [unwired: 2 in, 1 out]
              }
            }
          }
        }
        n90 = Get Date/Time In Seconds() -> (seconds since 1Jan1904=w150:timestamp)
        n91 = global read "断电保存变量.vi" "溶解氧参数"() -> (w152:T4)
        n92 = Bundle By Name(cluster=w152, "空白校准时间"=w150, "标样校准时间"=w150) -> (w151:T4)
        n93 = global write "断电保存变量.vi" "溶解氧参数"(w151) -> ()
        n94 = call "Add State to Queue.vi"("State(s) In (\"\")"="init: all\nCal: Over\nidle" ("State(s) In (\"\")")) -> ("States Out"=w156:string)  [unwired: 14 in]
        n95 = global read "多参数全局变量.vi" "多参数编号"() -> (w162:string)
        n96 = Format Into String(format string="编号：%s\n参数：%s\n信息：%s\n电极零点=%#.2f%%，电极斜率=%#.2f%%" ("格式字符串"), w162, w161, w158, w155, w154) -> (resulting string=w159:string)  [unwired: 2 in, 1 out]
        n97 = One Button Dialog(message=w159) -> ()  [unwired: 1 in, 1 out]
        n98 = call "校准日志.vi"("table"="校准记录", "日志信息"=w159) -> ()  [unwired: 9 in, 1 out]
      }
      frame "Cal: Over" {
        n99 = global read "多参数全局变量.vi" "校准运行状态"() -> (w184:T5)
        n100 = Bundle By Name(cluster=w184, "DO"=FALSE) -> (w185:T5)
        n101 = global write "多参数全局变量.vi" "校准运行状态"(w185) -> ()
      }
      frame "idle", Default {
        n102 = event shown="[5] \"滤波设定\": 值改变" {
          selector: _ -> [_ _ _ _ _ _ _ _ _ _ _]
          dyn-events: _ -> [_ _ _ _ _ _ _ _ _ _ _]
          timeout: 10 -> [_ _ _ _ _ _ _ _ _ _ _]
          tunnel: [_ _ _ _ w239 w244 w251 w257 _ _ _] -> _
          tunnel: w196 -> [w212 w216 w221 w233 w238 w247 w250 w256 w264 w275 _]
          tunnel: [w211 w215 w222 w234 w242 w248 w254 w260 w263 w274 w277] -> w195
          tunnel: [w210 w213 w223 w235 w243 w249 w255 w261 w262 w272 w278] -> w194
          tunnel: w193 -> [w210 w213 w223 w235 w243 w249 w255 w261 w262 w272 w278]
          event Timeout {
            n103 = event-data() -> ()  [unwired: 1 in, 3 out]
            n104 = global read "国弘过程全局变量.vi" "DO"() -> (w198:T2)
            n105 = Unbundle By Name(w198) -> ("命令滤波设定"=→"滤波设定":u16, "溶解氧电极零点"=→"电极零点":sgl, "溶解氧电极斜率"=→"电极斜率":sgl, "大气压补偿值"=→"气压补偿值":sgl, "盐度补偿值"=→"盐度补偿值":sgl, "溶解氧偏移修正值"=→"偏移值补偿":sgl, "溶解氧饱和度值"=→"饱和度值":sgl, "溶解氧测量值"=→"测量读值":sgl)
            n106 = global read "多参数全局变量.vi" "DO通讯状态"() -> (w209:bool)
            n107 = property on="通讯状态" class="Str"("Blinking"=TRUE ("闪烁"), "Text.BG Color"=u32 16711680, "Visible"=w209) -> ()  [unwired: 2 in, 2 out]
            n108 = call "Add State to Queue.vi"("State(s) In (\"\")"=w212) -> ("States Out"=w211:string)  [unwired: 14 in]
            "通讯状态" <- "通讯异常" ("当前串口")
          }
          event "校准模式": Value Change {
            n109 = event-data() -> ()  [unwired: 1 in, 6 out]
            n110 = call "Add State to Queue.vi"("State(s) In (\"\")"=w216, "State(s) At Back (\"\")"="init: all\nidle" ("State(s) In (\"\")")) -> ("States Out"=w215:string)  [unwired: 13 in]
          }
          event "气压补偿值", "偏移值补偿", "滤波设定": Mouse Down {
            n111 = event-data() -> ("CtlRef"=w220:refnum<vi>)  [unwired: 1 in, 7 out]
            n112 = property class="DigNum (严格)"(reference=w220) -> (reference out=w217:refnum<vi>, "Value"=w218:dbl)  [unwired: 1 in, 1 out]
            n113 = call "数字键盘.vi"("OldNumber"=w218) -> ("NewNumber"=w219:dbl)  [unwired: 1 in]
            n114 = property class="DigNum (严格)"(reference=w217, "Val(Sgnl)"=w219) -> ()  [unwired: 1 in, 2 out]
            n115 = call "Add State to Queue.vi"("State(s) In (\"\")"=w221) -> ("States Out"=w222:string)  [unwired: 14 in]
          }
          event "盐度补偿值": Mouse Down {
            n116 = event-data() -> ("CtlRef"=w232:refnum<vi>)  [unwired: 1 in, 7 out]
            n117 = global read "断电保存变量.vi" "Cond"() -> (w224:bool)
            n118 = case shown="真" w224 {
              tunnel: [_ w236] -> w229
              frame False {
              }
              frame True {
                n119 = Two Button Dialog(message="是否使用系统测试值自动补偿" ("消息")) -> (T button?=w236:bool)  [unwired: 2 in]
              }
            }
            n120 = global read "多参数全局变量.vi" "盐度显示"() -> (w228:T6)
            n121 = Unbundle By Name(w228) -> ("测量值"=w227:sgl)
            n122 = property class="DigNum (严格)"(reference=w232) -> (reference out=w230:refnum<vi>, "Value"=w226:dbl)  [unwired: 1 in, 1 out]
            n123 = Select(t=w227, s=w229, f=w226) -> (s? t:f=w225:dbl)
            n124 = call "数字键盘.vi"("OldNumber"=w225) -> ("NewNumber"=w231:dbl)  [unwired: 1 in]
            n125 = property class="DigNum (严格)"(reference=w230, "Val(Sgnl)"=w231) -> ()  [unwired: 1 in, 2 out]
            n126 = call "Add State to Queue.vi"("State(s) In (\"\")"=w233) -> ("States Out"=w234:string)  [unwired: 14 in]
          }
          event "盐度补偿值": Value Change {
            n127 = event-data() -> ("NewVal"=w240:dbl)  [unwired: 1 in, 5 out]
            n128 = global read "多参数全局变量.vi" "MB session in"() -> (w241:refnum<class "MB_Master.lvclass">)
            n129 = call "0008H_DO_盐度补偿值写入.vi"("数值"=w240, "MB session in"=w241) -> ("error out"=w239:errorcluster)  [unwired: 8 in, 1 out]
            n130 = call "Add State to Queue.vi"("State(s) In (\"\")"=w238) -> ("States Out"=w242:string)  [unwired: 14 in]
          }
          event "滤波设定": Value Change {
            n131 = event-data() -> ("NewVal"=w245:dbl)  [unwired: 1 in, 5 out]
            n132 = global read "多参数全局变量.vi" "MB session in"() -> (w246:refnum<class "MB_Master.lvclass">)
            n133 = call "0027H_DO_数位滤波设定写入.vi"("数值"=w245, "MB session in"=w246) -> ("error out"=w244:errorcluster)  [unwired: 8 in, 1 out]
            n134 = call "Add State to Queue.vi"("State(s) In (\"\")"=w247) -> ("States Out"=w248:string)  [unwired: 14 in]
          }
          event "气压补偿值": Value Change {
            n135 = event-data() -> ("NewVal"=w252:dbl)  [unwired: 1 in, 5 out]
            n136 = global read "多参数全局变量.vi" "MB session in"() -> (w253:refnum<class "MB_Master.lvclass">)
            n137 = call "000AH_DO_大气压补偿值写入.vi"("数值"=w252, "MB session in"=w253) -> ("error out"=w251:errorcluster)  [unwired: 8 in, 1 out]
            n138 = call "Add State to Queue.vi"("State(s) In (\"\")"=w250) -> ("States Out"=w254:string)  [unwired: 14 in]
          }
          event "偏移值补偿": Value Change {
            n139 = event-data() -> ("NewVal"=w258:dbl)  [unwired: 1 in, 5 out]
            n140 = global read "多参数全局变量.vi" "MB session in"() -> (w259:refnum<class "MB_Master.lvclass">)
            n141 = call "000CH_DO_DO偏移修正值写入.vi"("数值"=w258, "MB session in"=w259) -> ("error out"=w257:errorcluster)  [unwired: 8 in, 1 out]
            n142 = call "Add State to Queue.vi"("State(s) In (\"\")"=w256) -> ("States Out"=w260:string)  [unwired: 14 in]
          }
          event "刷新按钮": Value Change {
            n143 = event-data() -> ()  [unwired: 1 in, 6 out]
            n144 = call "Add State to Queue.vi"("State(s) In (\"\")"=w264) -> ("States Out"=w263:string)  [unwired: 14 in]
            n145 = Two Button Dialog(message="请再次确实是否恢复出厂设置！" ("消息")) -> (T button?=w266:bool)  [unwired: 2 in]
            n146 = case shown="真" w266 {
              frame False {
              }
              frame True {
                w267 = u16 33 items=["Factory Reset"=33] ("数值")
                n147 = global read "多参数全局变量.vi" "MB session in"() -> (w268:refnum<class "MB_Master.lvclass">)
                n148 = call "0026H_DO_命令寄存器写入.vi"("数值"=w267, "MB session in"=w268) -> ()  [unwired: 8 in, 2 out]
              }
            }
          }
          event "校准启动": Value Change {
            n149 = event-data() -> ()  [unwired: 1 in, 6 out]
            n150 = global read "多参数全局变量.vi" "校准运行状态"() -> (w270:T5)
            n151 = call "Add State to Queue.vi"("State(s) In (\"\")"=w275, "State(s) At Back (\"\")"="init: all\nCal: Place standard solution\n Cal: Calibration process\nidle" ("State(s) In (\"\")")) -> ("States Out"=w274:string)  [unwired: 13 in]
            n152 = Bundle By Name(cluster=w270, "DO"=TRUE) -> (w271:T5)
            n153 = global write "多参数全局变量.vi" "校准运行状态"(w271) -> ()
          }
          event "校准停止": Value Change {
            n154 = event-data() -> ()  [unwired: 1 in, 6 out]
            n155 = call "Add State to Queue.vi"("State(s) In (\"\")"="init: all\nCal: Over\nidle" ("State(s) In (\"\")")) -> ("States Out"=w277:string)  [unwired: 14 in]
          }
        }
      }
    }
  }
  n156 = while {
    stop <- FALSE stop-if-true
    n157 = global read "多参数全局变量.vi" "权限"() -> (w282:enum16{"一级权限", "二级权限", "三级权限"})
    n158 = Wait (ms)(milliseconds to wait=u32 1000 ("等待时间（毫秒）")) -> ()  [unwired: 1 out]
    n159 = Not Equal?(x=w282, y=enum16{"一级权限", "二级权限", "三级权限"}."一级权限") -> (x != y?=w279:bool)
    n160 = property on="偏移值补偿" class="DigNum (严格)"("Visible"=w279) -> ()  [unwired: 2 in, 2 out]
    n161 = property on="滤波设定" class="DigNum (严格)"("Visible"=w279) -> ()  [unwired: 2 in, 2 out]
  }
